vi "k26xx_I-V_sweep_simple.vi"() -> ()   [LabVIEW 2017]
uses:
  Keithley_26xx/Public/Channel.ctl
  <vilib>/Analysis/1siggen.llb/Ramp Pattern by Samples.vi
  Keithley_26xx/Keithley 2600 Series.lvlib
  <vilib>/Analysis/NI_AALBase.lvlib
panel:
  out "error out":errorcluster
  in  "# Steps":u32=101
  out "Comp?":bool=TRUE caption="Compliance?"
  in  "Stop Button":bool
  out "XY Graph":cluster{dbl[], dbl[]}(graph)={[-0.0906631, -0.0920705, 0.554765, 1.27002, 1.96684, 2.7166, 3.48363, 4.26629, 5.09515, 6.01407, 6.87621, 7.64287, 8.49814, 9.21752, 9.94246], [0.000104785, 0.000102878, 0.00106434, 0.00205982, 0.00305593, 0.00405455, 0.00505181, 0.00604653, 0.00703088, 0.0080413, 0.00904946, 0.0100603, 0.0110564, 0.0120458, 0.0129968]}
  out "I, V":string="1.29968e-02, 9.94246e+00\n" caption="Measured Values:  I, V"
  in  "Measure Delay (s)":dbl=0.01 min=0.0 step=0.1 format="%#_6p"
  in  "Sense Type":enum32{"2 Wire", "4 Wire", "Calibration"}(ring)=enum."4 Wire"
  in  "NPLC":dbl=1.0
  in  "Sweep Type (i)":enum32{"Current", "Voltage"}(ring) caption="Sweep Type"
  in  "Channel (Channel A)":T1
  in  "error":errorcluster
  in  "Sweep End":dbl=0.1
  in  "Compliance":dbl=10.0 format="%#_6p"
  in  "Sweep Start":dbl
  in  "SMU":refnum<visa-resource-name>="GPIB0::22::INSTR"
  # "Keithley 26xx I-V sweep with variable delay between measurements.  (Note that NPLC will affect delay also!)\n Craig Storey, 2018/10/30"
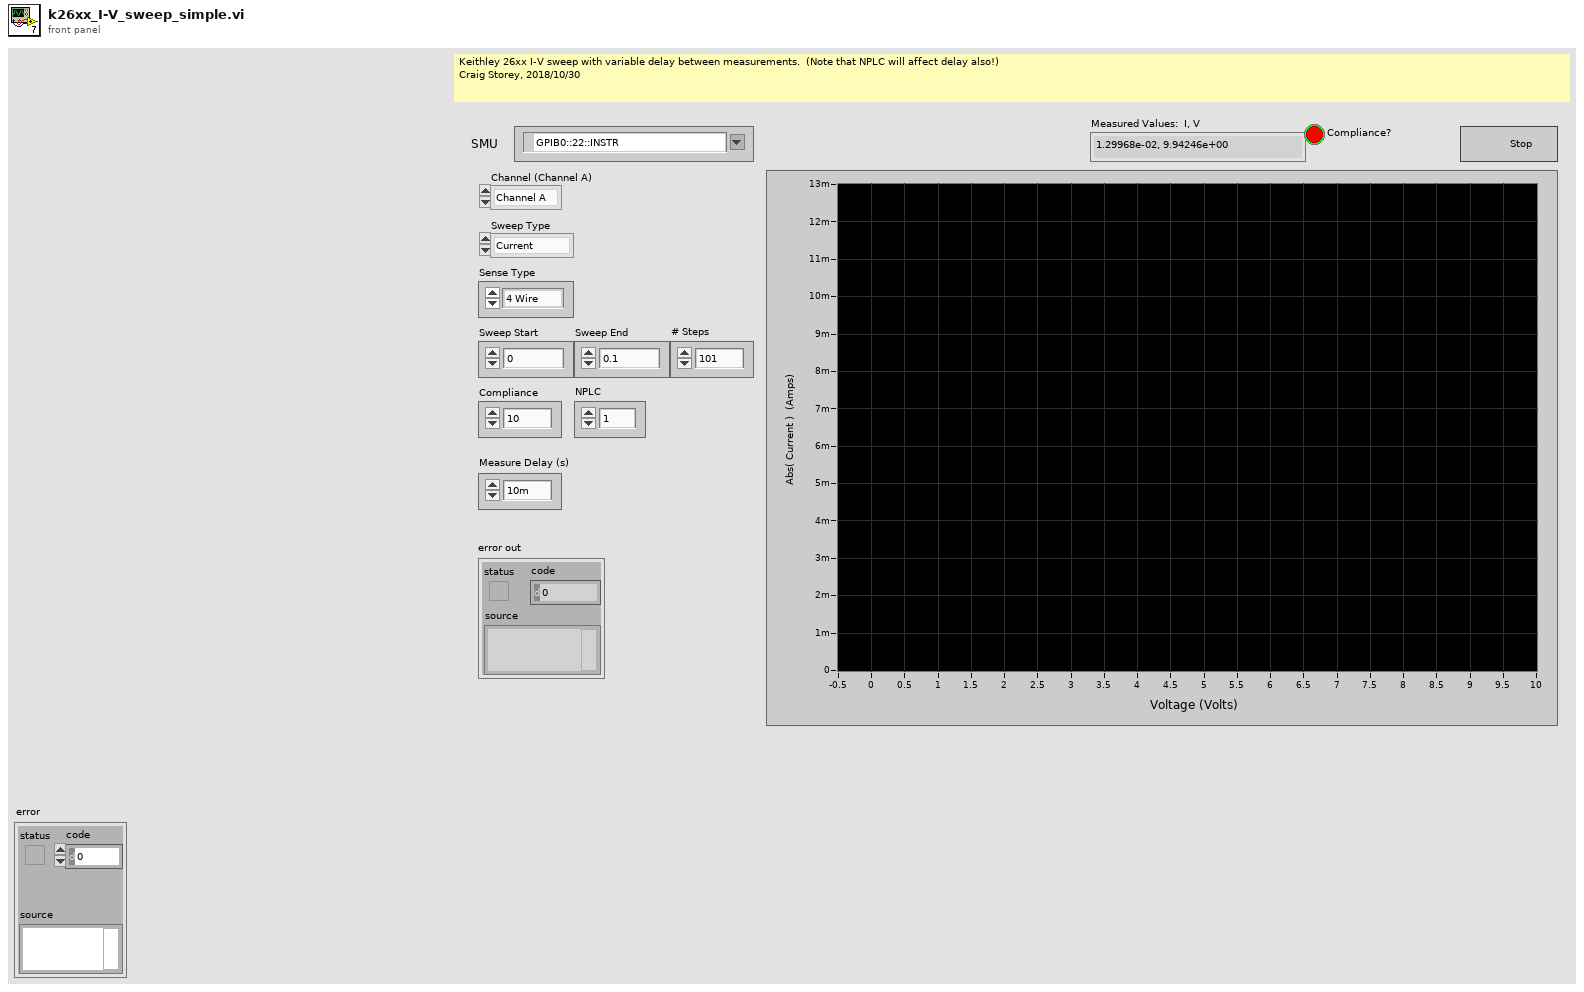
[diagram p1: front panel]
types:
  T1 = typedef "Keithley 2600 Series.lvlib/Channel.ctl" = enum32{"Channel A", "Channel B"}
  T2 = enum32{"Current", "Voltage", "IV", "Resistance", "Power"}
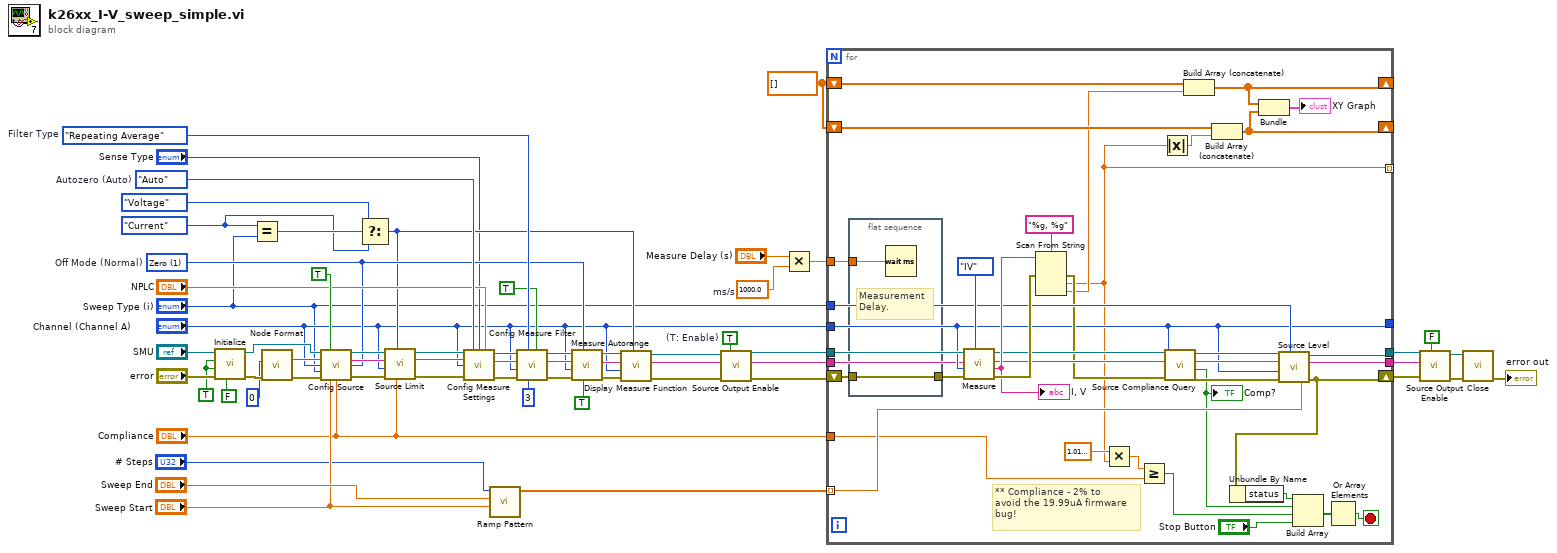
[diagram p0: block diagram]
diagram:
  w1 = dbl[] []
  w11 = 1000.0  # ms/s
  w25 = TRUE  # (T: Enable)
  w48 = enum32{"Moving Average", "Repeating Average"}."Repeating Average"  # Filter Type
  w37 = u16 1 items=["Normal", "Zero", "High Z"]  # Off Mode (Normal)
  w54 = enum32{"Off", "Once", "Auto"}."Auto"  # Autozero (Auto)
  w56 = enum32{"Current", "Voltage"}."Current" ("x")
  w35 = TRUE ("Error Query (False)")
  n1 = call "Initialize.vi"("Reset (True)"=FALSE, "error in (no error)"="error", "Error Query (False)"=w35, "ID Query (True)"=w35, "VISA resource name"="SMU") -> ("error out"=w60:errorcluster, "VISA resource name out"=w32:refnum<visa-resource-name>)  [unwired: 1 in, 4 out]
  n2 = Equal?(x=w56, y="Sweep Type (i)") -> (x = y?=w57:bool)
  n3 = call "Node Format.vi"("error in"=w60, "Node (0-64)"=i8 0) -> ("error out"=w33:errorcluster, "Formatted Node"=w31:string)  [unwired: 8 out]
  n4 = call "Config Source.vi"("VISA resource name"=w32, "Autorange (On)"=TRUE, "Node In"=w31, "Channel (Channel A)"="Channel (Channel A)", "Off Mode (Normal)"=w37, "Function (Current)"="Sweep Type (i)", "error in"=w33, "Level (0.000)"="Sweep Start", "Limit (0.1)"="Compliance") -> ("VISA resource name out"=w39:refnum<visa-resource-name>, "Node Out"=w40:string, "error out"=w38:errorcluster)  [unwired: 2 in, 2 out]
  n5 = Select(t=enum32{"Current", "Voltage"}."Voltage" ("x"), s=w57, f=w56) -> (s? t:f=w27:enum32{"Current", "Voltage"})
  n6 = call "Source Limit.vi"("Limit (0.000)"="Compliance", "Function (Current)"=w27, "error in (no error)"=w38, "Channel (Channel A)"="Channel (Channel A)", "Node In"=w40, "VISA resource name"=w39) -> ("error out"=w43:errorcluster, "Node Out"=w42:string, "VISA resource name out"=w41:refnum<visa-resource-name>)  [unwired: 2 in, 1 out]
  n7 = call "Config Measure Settings.vi"("VISA resource name"=w41, "Autozero (Auto)"=w54, "Sense (2 Wire)"="Sense Type", "NPLC (1.000)"="NPLC", "Node In"=w42, "Channel (Channel A)"="Channel (Channel A)", "error in"=w43) -> ("VISA resource name out"=w49:refnum<visa-resource-name>, "Node Out"=w50:string, "error out"=w51:errorcluster)  [unwired: 5 in, 1 out]
  n8 = call-poly <vilib>:"Ramp Pattern.vi"("start"="Sweep Start", "end"="Sweep End", "samples"="# Steps") -> ("Ramp Pattern"=w14:dbl[])  [unwired: 7 in, 1 out]
  n9 = call "Config Measure Filter.vi"("On/Off (Off)"=TRUE, "Count (1)"=3, "Filter Type (Moving Average)"=w48, "error in"=w51, "Channel (Channel A)"="Channel (Channel A)", "Node In"=w50, "VISA resource name"=w49) -> ("error out"=w46:errorcluster, "Node Out"=w45:string, "VISA resource name out"=w44:refnum<visa-resource-name>)  [unwired: 1 in, 1 out]
  n10 = call "Measure Autorange.vi"("Autorange (On)"=TRUE, "Function (Current)"=w37, "error in (no error)"=w46, "Channel (Channel A)"="Channel (Channel A)", "Node In"=w45, "VISA resource name"=w44) -> ("error out"=w30:errorcluster, "Node Out"=w29:string, "VISA resource name out"=w28:refnum<visa-resource-name>)  [unwired: 2 in, 1 out]
  n11 = call "Display Measure Function.vi"("Function (Current)"=w27, "error in (no error)"=w30, "Channel (Channel A)"="Channel (Channel A)", "Node In"=w29, "VISA resource name"=w28) -> ("error out"=w23:errorcluster, "Node Out"=w19:string, "VISA resource name out"=w24:refnum<visa-resource-name>)  [unwired: 3 in, 1 out]
  n12 = call "Source Output Enable.vi"("Output (Off)"=w25, "error in (no error)"=w23, "Node In"=w19, "VISA resource name"=w24) -> ("error out"=w10:errorcluster, "Node Out"=w18:string, "VISA resource name out"=w20:refnum<visa-resource-name>)  [unwired: 1 in, 4 out]
  n13 = Multiply(x="Measure Delay (s)", y=w11) -> (x*y=w13:dbl)
  n14 = for {
    shift-right: [w92] -> w6
    shift-left: w10 -> [w65]
    tunnel: w20 -> [w94]
    tunnel: [w91] -> w4
    tunnel: w13 -> [w100]
    tunnel: "Channel (Channel A)" -> [w79]
    tunnel: [w90] -> w5
    tunnel: [w79] -> _
    tunnel: "Sweep Type (i)" -> [w86]
    shift-right: [w72] -> _
    shift-left: w1 -> [w77]
    shift-right: [w73] -> _
    shift-left: w1 -> [w76]
    tunnel: w18 -> [w71]
    tunnel: w14 -> [w70] mode=indexing
    tunnel: [w69] -> _ mode=indexing
    tunnel: "Compliance" -> [w63]
    stop <- w99 stop-if-true
    # "** Compliance - 2% to\navoid the 19.99uA firmware\nbug!"
    n15 = flat-sequence {
      tunnel: w100 -> [w102]
      tunnel: [w101] -> w66
      tunnel: w65 -> [w101]
      frame #0 {
        # "Measurement\nDelay."
        n16 = Wait (ms)(milliseconds to wait=w102) -> ()  [unwired: 1 out]
      }
    }
    n17 = call "Measure.vi"("Function (Current)"=T2."IV", "error in (no error)"=w66, "Channel (Channel A)"=w79, "Node In"=w71, "VISA resource name"=w94) -> ("error out"=w89:errorcluster, "Output"=w87:string, "Node Out"=w83:string, "VISA resource name out"=w82:refnum<visa-resource-name>)  [unwired: 2 in, 1 out]
    "I, V" <- w87
    n18 = Scan From String(format string="%g, %g", input string=w87, error in=w89) -> (error out=w80:errorcluster, output 1=w69:dbl, output 2=w75:dbl)  [unwired: 3 in, 2 out]
    n19 = Multiply(x=sgl 1.02 ("y"), y=w69) -> (x*y=w64:dbl)
    n20 = Greater Or Equal?(x=w64, y=w63) -> (x >= y?=w96:bool)
    n21 = Absolute Value(x=w69) -> (abs(x)=w74:dbl)
    n22 = call "Source Compliance Query.vi"("error in (no error)"=w80, "Channel (Channel A)"=w79, "Node In"=w83, "VISA resource name"=w82) -> ("error out"=w85:errorcluster, "Compliance"=w67:bool, "Node Out"=w84:string, "VISA resource name out"=w81:refnum<visa-resource-name>)  [unwired: 3 in, 1 out]
    "Comp?" <- w67
    n23 = Build Array (concatenate)(w77, w75) -> (w72:dbl[])
    n24 = Build Array (concatenate)(w76, w74) -> (w73:dbl[])
    n25 = Bundle(w72, w73) -> (→"XY Graph":cluster{dbl[], dbl[]})  [unwired: 1 in]
    n26 = call "Source Level.vi"("Level (0.000)"=w70, "Function (Current)"=w86, "error in (no error)"=w85, "Channel (Channel A)"=w79, "Node In"=w84, "VISA resource name"=w81) -> ("error out"=w92:errorcluster, "Node Out"=w90:string, "VISA resource name out"=w91:refnum<visa-resource-name>)  [unwired: 3 out]
    n27 = Unbundle By Name(w92) -> ("status"=w68:bool)
    n28 = Build Array(w68, w67, w96, "Stop Button") -> (w98:bool[])
    n29 = Or Array Elements(Boolean array=w98) -> (logical OR=w99:bool)
  }
  n30 = call "Source Output Enable.vi"("Output (Off)"=FALSE ("Enable Output (T: Enable)"), "error in (no error)"=w6, "Node In"=w5, "VISA resource name"=w4) -> ("error out"=w8:errorcluster, "VISA resource name out"=w9:refnum<visa-resource-name>)  [unwired: 1 in, 5 out]
  n31 = call "Close.vi"("error in (no error)"=w8, "VISA resource name"=w9) -> ("error out"=→"error out":errorcluster)  [unwired: 9 out]
